vi "calculate trace.vi"() -> ()   [LabVIEW 2012]
uses:
  <vilib>/Utility/file.llb/Write To Spreadsheet File (DBL).vi
  <vilib>/Utility/file.llb/Read From Spreadsheet File (DBL).vi
  <vilib>/Analysis/baseanly.llb/Mean (DBL).vi
  <vilib>/Analysis/NI_AALBase.lvlib
panel:
  in  "txt folder Path":path
  out "error out":errorcluster
  in  "error in (no error)":errorcluster
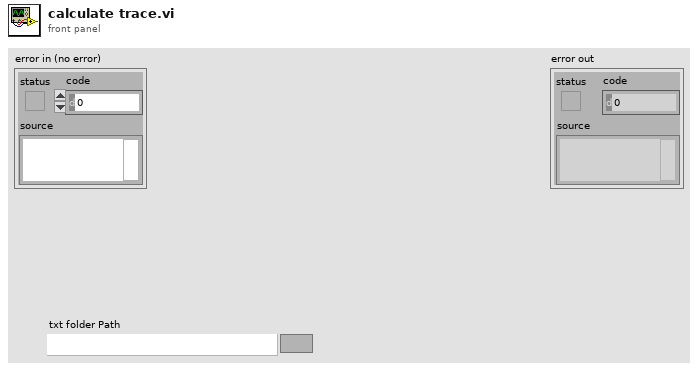
[diagram p1: front panel]
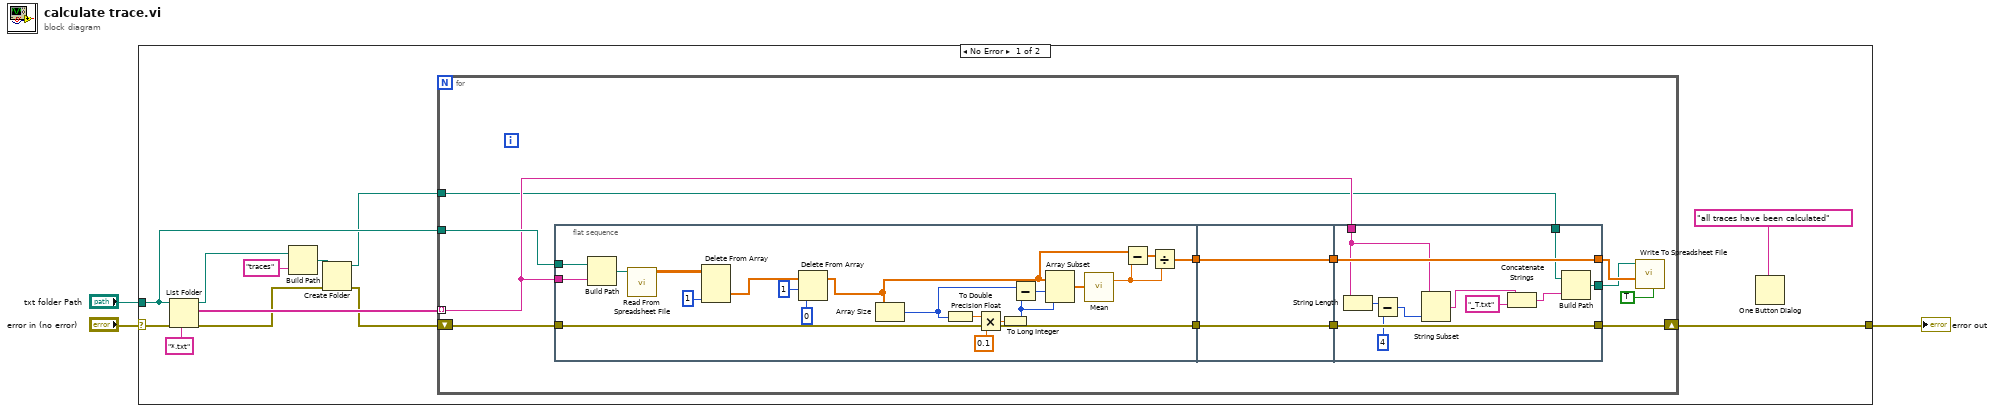
[diagram p0: block diagram]
diagram:
  n1 = case shown="No Error" "error in (no error)" {
    selector: "error in (no error)" -> [w15 w61]
    tunnel: [w11 w61] -> w2
    tunnel: "txt folder Path" -> [w12 _]
    frame No Error {
      n2 = List Folder(path=w12, pattern="*.txt", error in=w15) -> (path out=w6:path, filenames=w13:string[], error out=w8:errorcluster)  [unwired: 1 in, 1 out]
      n3 = Build Path(base path=w6, name or relative path="traces") -> (appended path=w9:path)
      n4 = Create Folder(path (use dialog)=w9, error in=w8) -> (created path=w5:path, error out=w7:errorcluster)  [unwired: 1 in, 1 out]
      n5 = for {
        shift-right: [w26] -> w11
        shift-left: w7 -> [w27]
        tunnel: w13 -> [w20] mode=indexing
        tunnel: w12 -> [w24]
        tunnel: w5 -> [w17]
        n6 = flat-sequence {
          tunnel: w27 -> [w47]
          tunnel: [w47] -> w25
          tunnel: w20 -> [w37]
          tunnel: w24 -> [w36]
          tunnel: [w34] -> w23
          tunnel: w25 -> [w48]
          tunnel: w23 -> [w49]
          tunnel: [w48] -> w22
          tunnel: [w49] -> w21
          tunnel: [w59] -> w19
          tunnel: [w60] -> w26
          tunnel: w22 -> [w60]
          tunnel: w21 -> [w59]
          tunnel: w20 -> [w53]
          tunnel: [w52] -> w18
          tunnel: w17 -> [w51]
          frame #0 {
            n7 = Build Path(base path=w36, name or relative path=w37) -> (appended path=w38:path)
            n8 = call-poly <vilib>:"Read From Spreadsheet File.vi"("file path (dialog if empty)"=w38) -> ("all rows"=w33:dbl[][])  [unwired: 6 in, 4 out]
            n9 = Delete From Array(array=w33, index (col)=1 ("disabled index (col)")) -> (deleted portion=w31:dbl[])  [unwired: 2 in, 1 out]
            n10 = Delete From Array(array=w31, length=1, index=0) -> (array with subset deleted=w28:dbl[])  [unwired: 1 out]
            n11 = Array Size(array=w28) -> (size(s)=w41:i32)
            n12 = To Double Precision Float(number=w41) -> (double precision float=w39:dbl)
            n13 = Multiply(x=w39, y=0.1) -> (x*y=w40:dbl)
            n14 = To Long Integer(number=w40) -> (32bit integer=w42:i32)
            n15 = Subtract(x=w41, y=w42) -> (x-y=w43:i32)
            n16 = Array Subset(array=w28, index=w43, length=w42) -> (w44:dbl[])
            n17 = call-poly <vilib>:"Mean.vi"("X"=w44) -> ("mean"=w46:dbl)  [unwired: 1 out]
            n18 = Subtract(x=w28, y=w46) -> (x-y=w45:dbl[])
            n19 = Divide(x=w45, y=w46) -> (x/y=w34:dbl[])
          }
          frame #1 {
          }
          frame #2 {
            n20 = String Length(string=w53) -> (length=w56:i32)
            n21 = Subtract(x=w56, y=4) -> (x-y=w50:i32)
            n22 = String Subset(string=w53, length (rest)=w50) -> (substring=w55:string)  [unwired: 1 in]
            n23 = Concatenate Strings(w55, "_T.txt" ("string")) -> (w58:string)
            n24 = Build Path(base path=w51, name or relative path=w58) -> (appended path=w52:path)
          }
        }
        n25 = call-poly <vilib>:"Write To Spreadsheet File.vi"("transpose? (no:F)"=TRUE, "1D data"=w19, "file path (dialog if empty)"=w18) -> ()  [unwired: 5 in, 1 out]
      }
      n26 = One Button Dialog(message="all traces have been calculated") -> ()  [unwired: 1 in, 1 out]
    }
    frame Error {
    }
  }
  "error out" <- w2
